vi "MultiLineString_Create.vi"(0 "reference":refnum<class "MultiLineString.lvclass">, 1 "GAP":i32=3, 5 "error in (no error)":errorcluster) -> (14 "reference out":refnum<class "MultiLineString.lvclass">, 19 "error out":errorcluster)   [LabVIEW 2014, in "MultiLineString.lvclass"]
doc: "Creates and initializes a new MultiLineString object.\n\nThis object should be destroyed using a MultiLineString destructor VI.\n\n[GOOP 2.3]"
uses:
  <resource>/Framework/Providers/Open_GDS/UML/MultiLineString_class/MultiLineString.lvclass
  <resource>/Framework/Providers/Open_GDS/UML/MultiLineString_class/JustificationType.ctl
  <resource>/Framework/Providers/Open_GDS/UML/MultiLineString_class/SizeType.ctl
panel:
  # "The input reference should only\nbe wired when this method is called\nby a sub class constructor."
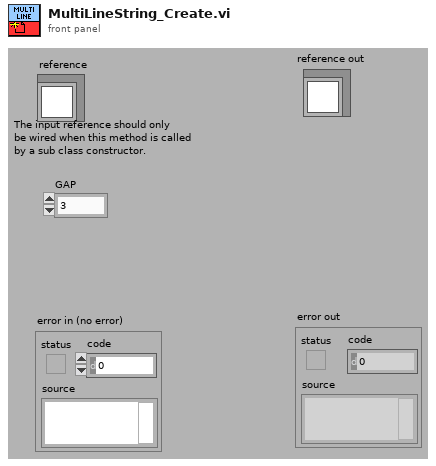
[diagram p1: front panel]
types:
  T1 = typedef "MultiLineString.lvclass/SizeType.ctl" = enum16{"LARGE", "NORMAL", "SMALL"}
  T2 = typedef "MultiLineString.lvclass/JustificationType.ctl" = enum16{"LEFT", "CENTER", "RIGHT"}
  T3 = typedef "MultiLineString.lvclass/ObjectAttributes.ctl" = cluster{"GAP":i32, "text":string, "justification":T2, "size":T1, "underlined":bool}
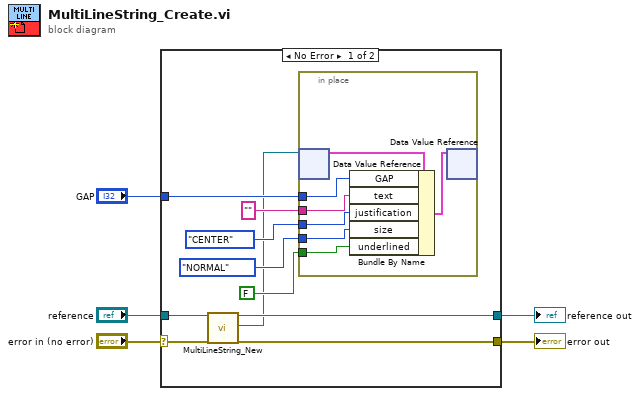
[diagram p0: block diagram]
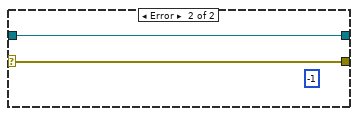
[diagram p2: hidden frame]
diagram:
  n1 = case shown="No Error" "error in (no error)" {
    selector: "error in (no error)" -> [w15 w24]
    tunnel: [w8 w23] -> w5
    tunnel: [w7 w24] -> w4
    tunnel: "reference" -> [w14 w23]
    tunnel: "GAP" -> [w13 _]
    frame No Error {
      n2 = call <resource>:"MultiLineString_New.vi"("reference in"=w14, "error in (no error)"=w15) -> ("reference out"=w8:refnum<class "MultiLineString.lvclass">, "DVRRefOut"=w6:refnum<data-value>, "error out"=w7:errorcluster)  [unwired: 3 in, 12 out]
      n3 = in-place {
        in-place-border: w13 -> [w21]
        in-place-border: "" ("text") -> [w20]
        in-place-border: JustificationType."CENTER" ("justification") -> [w19]
        in-place-border: SizeType."NORMAL" ("size") -> [w18]
        in-place-border: FALSE ("underlined") -> [w17]
        n4 = in-place-dvr #1(w6) -> (w22:T3)  [unwired: 1 out]
        n5 = Bundle By Name(cluster=w22, "GAP"=w21, "text"=w20, "justification"=w19, "size"=w18, "underlined"=w17) -> (w16:T3)
        n6 = in-place-dvr #1(w16) -> ()  [unwired: 2 out]
      }
    }
    frame Error {
      (unwired) -1 ("Nr of open handles")
    }
  }
  "error out" <- w4
  "reference out" <- w5
